vi "connect test.vi"() -> ()   [LabVIEW 2017]
uses:
  <vilib>/Plasmionique/MB Master/MB_Master_Serial/MB_Master_Serial.lvclass
  D:/Program Files (x86)/National Instruments/LabVIEW 2017/vi.lib/Plasmionique/MB Master/MB_Master/MB_Master.lvclass
  <vilib>/Plasmionique/MB Master/MB Master.lvlib
panel:
  out "Coils 2":bool[](array[boolean])
  out "Coils":bool[](array[boolean])
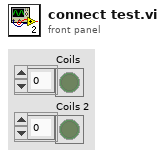
[diagram p1: front panel]
types:
  T1 = cluster{"baud rate (bps)":u32, "stop bits":u16, "parity":u16, "flow control":u16, "timeout":u32, "retries":i32}
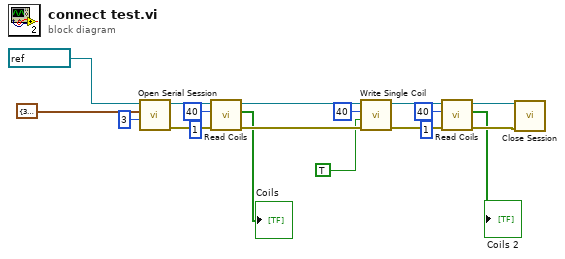
[diagram p0: block diagram]
diagram:
  n1 = call <vilib>:"Open Serial Session.vi"("Slave ID"=u8 3, "Serial Config"=T1 {"baud rate (bps)"=38400, "stop bits"=10, "parity"=0, "flow control"=0, "timeout"=1000, "retries"=1}, "VISA Resource"=refnum<visa-resource-name> "COM9") -> ("Error out"=w9:errorcluster, "MB_Serial session"=w8:refnum<class "MB_Master_Serial.lvclass">)  [unwired: 7 in]
  n2 = call <vilib>:"Read Coils.vi"("error in (no error)"=w9, "quantity"=u16 1, "starting address"=u16 40, "MB session in"=w8) -> ("error out"=w18:errorcluster, "Coils"=→"Coils":bool[], "MB session out"=w19:refnum<class "MB_Master_Serial.lvclass">)  [unwired: 5 in]
  n3 = call <vilib>:"Write Single Coil.vi"("error in (no error)"=w18, "value"=TRUE, "address"=u16 40, "MB session in"=w19) -> ("error out"=w13:errorcluster, "MB session out"=w12:refnum<class "MB_Master_Serial.lvclass">)  [unwired: 6 in]
  n4 = call <vilib>:"Read Coils.vi"("error in (no error)"=w13, "quantity"=u16 1, "starting address"=u16 40, "MB session in"=w12) -> ("error out"=w15:errorcluster, "Coils"=→"Coils 2":bool[], "MB session out"=w14:refnum<class "MB_Master_Serial.lvclass">)  [unwired: 5 in]
  n5 = call-dynamic "Close Session.vi"("error in (no error)"=w15, "MB_Serial session"=w14) -> ()  [unwired: 9 in, 1 out]
